vi "Get Control Data.vi"(8 "error in (no error)":errorcluster, 11 "VI Ref":refnum<vi>) -> (0 "error out":errorcluster, 2 "Control Data":T1[](array[typedef]), 3 "VI Ref out":refnum<vi>)   [LabVIEW 2023, in "VI Properties Editor.lvlib"]
doc: "Gets all control data for <B>VI Ref</B>."
uses:
  VI Properties Editor.lvlib
  CTLs/Control Properties.ctl
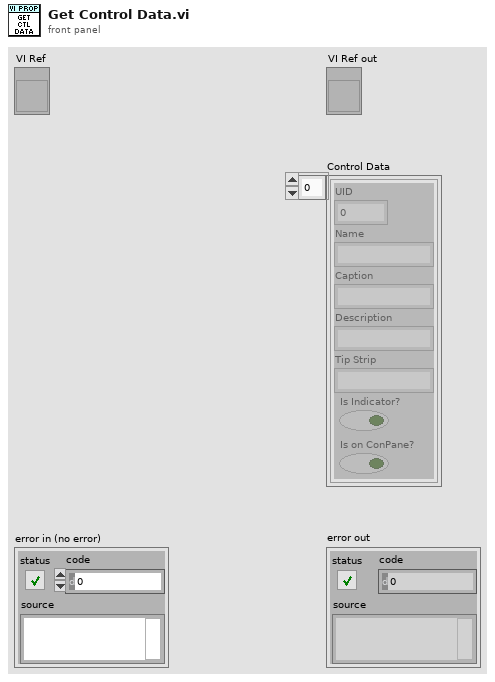
[diagram p1: front panel]
types:
  T1 = typedef "VI Properties Editor.lvlib/Control Properties.ctl" = cluster{"UID":i32, "Name":string, "Caption":string, "Description":string, "Tip Strip":string, "Is Indicator?":bool, "Is on ConPane?":bool}
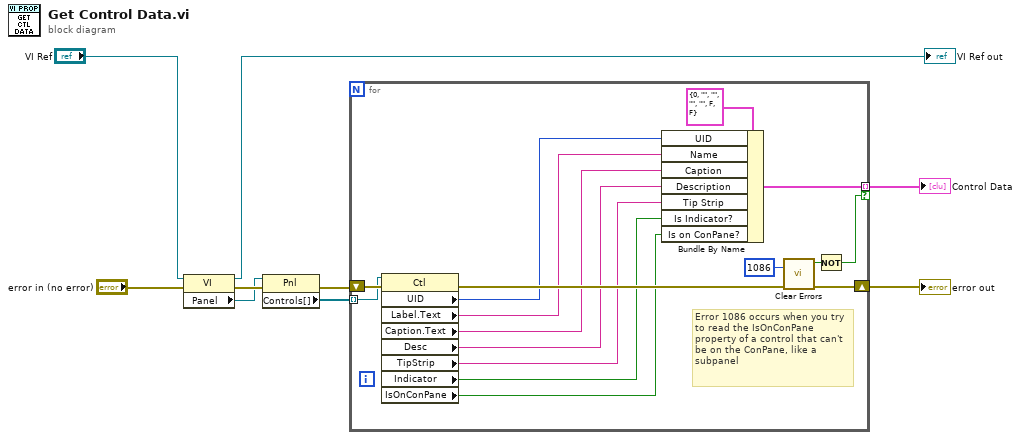
[diagram p0: block diagram]
diagram:
  n1 = property class="VI"(reference="VI Ref", error in="error in (no error)") -> (reference out=→"VI Ref out":refnum<vi>, error out=w4:errorcluster, "Panel"=w3:refnum<vi>)
  n2 = property class="Pnl"(reference=w3, error in=w4) -> (error out=w9:errorcluster, "Controls[]"=w8:refnum<vi>[])  [unwired: 1 out]
  n3 = for {
    tunnel: w8 -> [w23] mode=indexing
    shift-right: [w15] -> w7
    shift-left: w9 -> [w25]
    tunnel: [w20] -> w5 mode=indexing if=w13
    # "Error 1086 occurs when you try to read the IsOnConPane property of a control that can't be on the ConPane, like a subpanel"
    n4 = property class="Ctl"(reference=w23, error in=w25) -> (error out=w24:errorcluster, "UID"=w17:i32, "Label.Text"=w19:string, "Caption.Text"=w11:string, "Desc"=w10:string, "TipStrip"=w21:string, "Indicator"=w18:bool, "IsOnConPane"=w16:bool)  [unwired: 1 out]
    n5 = Bundle By Name(cluster=T1 {"UID"=0, "Name"="", "Caption"="", "Description"="", "Tip Strip"="", "Is Indicator?"=FALSE, "Is on ConPane?"=FALSE} ("Control Properties"), "UID"=w17, "Name"=w19, "Caption"=w11, "Description"=w10, "Tip Strip"=w21, "Is Indicator?"=w18, "Is on ConPane?"=w16) -> (w20:T1)
    n6 = call <vilib>:"Clear Errors.vi"("error in (no error)"=w24, "specific error code to clear (0: all)"=1086) -> ("error out"=w15:errorcluster, "specific error cleared?"=w14:bool)  [unwired: 4 in]
    n7 = Not(x=w14) -> (.not. x?=w13:bool)
  }
  "error out" <- w7
  "Control Data" <- w5
